vi "Link Parameters.vi"(8 "error in (no error)":errorcluster, 11 "Bus Controller in":refnum<class "Bus Controller.lvclass">) -> (0 "error out":errorcluster, 3 "Bus Controller out":refnum<class "Bus Controller.lvclass">)   [LabVIEW 2020, in "BCI-1553 API.lvlib" / "Bus Controller.lvclass"]
doc: "Populates the Parameter Read and Write tables with all the parameters in the message list contained in the Major Frame. These tables are used for quickly finding and accessing the data fields on the Board component memory."
uses:
  Bus Controller.lvclass
  C:/Users/MattJ/Desktop/git/bci-1553-labview-api/src/1553 SubComponent/1553 SubComponent.lvclass
  Bus Controller.lvclass/Bus Controller.ctl
  Dependencies/Registry/Registry.lvclass/Registry.ctl
  <vilib>/Utility/error.llb/Clear Errors.vi
  Dependencies/Registry/Registry.lvclass
  Frames & Messages/Major Frame/Major Frame.lvclass
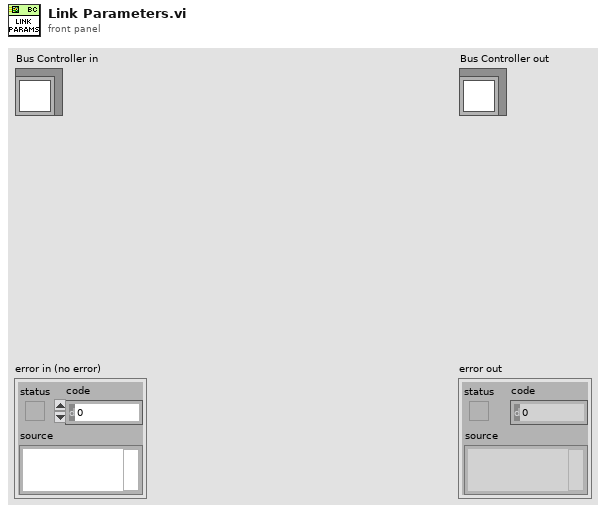
[diagram p1: front panel]
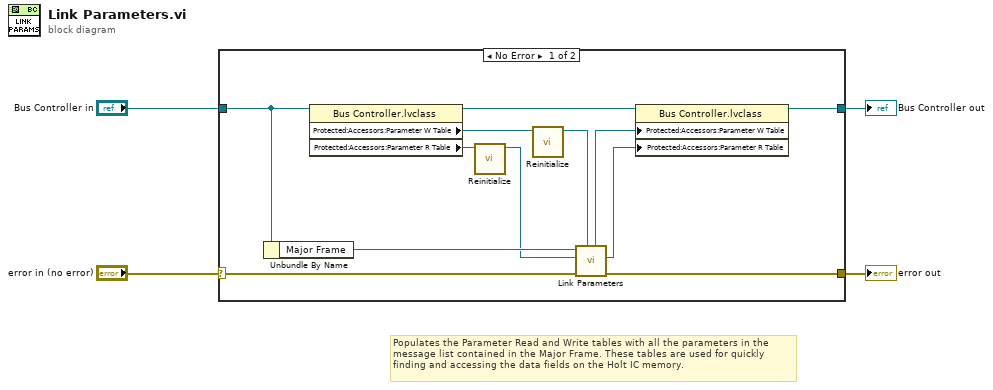
[diagram p0: block diagram]
diagram:
  # "Populates the Parameter Read and Write tables with all the parameters in the\nmessage list contained in the Major Frame. These tables are used for quickly\nfinding and accessing the data fields on the Holt IC memory."
  n1 = case shown="No Error" "error in (no error)" {
    selector: "error in (no error)" -> [w11 w18]
    tunnel: [w10 w18] -> w3
    tunnel: [w14 w17] -> w1
    tunnel: "Bus Controller in" -> [w9 w17]
    frame No Error {
      n2 = Unbundle By Name(w9) -> ("Major Frame"=w16:refnum<class "Major Frame.lvclass">)
      n3 = property class="Bus Controller.lvclass"(reference=w9) -> (reference out=w15:refnum<class "Bus Controller.lvclass">, "Protected:Accessors:Parameter W Table"=w6:refnum<class "Registry.lvclass">, "Protected:Accessors:Parameter R Table"=w8:refnum<class "Registry.lvclass">)  [unwired: 1 in, 1 out]
      n4 = call "Reinitialize.vi"("Registry in"=w8) -> ("Registry out"=w7:refnum<class "Registry.lvclass">)  [unwired: 9 in, 1 out]
      n5 = call "Reinitialize.vi"("Registry in"=w6) -> ("Registry out"=w5:refnum<class "Registry.lvclass">)  [unwired: 9 in, 1 out]
      n6 = call-dynamic "Link Parameters.vi"("Parameter W Table in"=w5, "error in (no error)"=w11, "Parameter R Table in"=w7, "Major Frame in"=w16) -> ("error out"=w10:errorcluster, "Parameter R Table out"=w12:refnum<class "Registry.lvclass">, "Parameter W Table out"=w13:refnum<class "Registry.lvclass">)  [unwired: 5 in]
      n7 = property class="Bus Controller.lvclass"(reference=w15, "Protected:Accessors:Parameter W Table"=w13, "Protected:Accessors:Parameter R Table"=w12) -> (reference out=w14:refnum<class "Bus Controller.lvclass">)  [unwired: 1 in, 1 out]
    }
    frame Error {
    }
  }
  "error out" <- w3
  "Bus Controller out" <- w1
